vi "Execute.vi"(8 "error in":errorcluster, 11 "O3 Valve Step in":refnum<class "O3 Valve Step.lvclass">) -> (0 "error out":errorcluster, 1 "Next Step?":bool, 2 "MSG":string, 3 "O3 Valve Step out":refnum<class "O3 Valve Step.lvclass">)   [LabVIEW 2016, in "Controller.lvlib" / "O3 Valve Step.lvclass"]
uses:
  O3 Valve Step.lvclass
  C:/Program Files (x86)/National Instruments/LabVIEW 2016/vi.lib/MSR Consulting, LLC/General Reuse/Sequence/STEPS/LEAVES/Switch/Switch Step.lvclass
  Messages/Update O3 Valve State MSG/Update O3 Valve State MSG.lvclass
  G:/sw_repo/For Builds/Nicholas/Controller/Messages/Generic Boolean MSG/Generic Boolean Message.lvclass
  C:/Program Files (x86)/National Instruments/LabVIEW 2016/vi.lib/ActorFramework/Message/Message.lvclass
  Messages/Generic Boolean MSG/Generic Boolean Message.lvclass/Generic Boolean Message.ctl
  <vilib>/ActorFramework/Message Enqueuer/Message Enqueuer.lvclass/Message Enqueuer.ctl
  Messages/Generic Boolean MSG/Write Bool.vi
  <vilib>/ActorFramework/Message Priority Queue/Priority Enqueue.vi
  gController.lvclass
  <vilib>/ActorFramework/Message Enqueuer/Message Enqueuer.lvclass
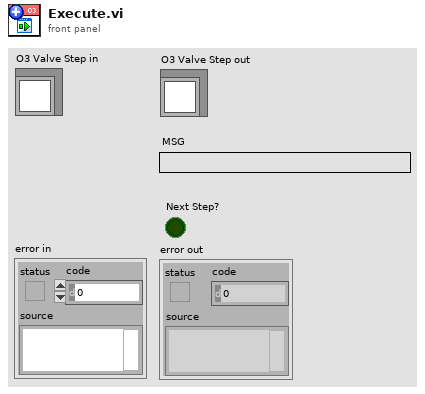
[diagram p1: front panel]
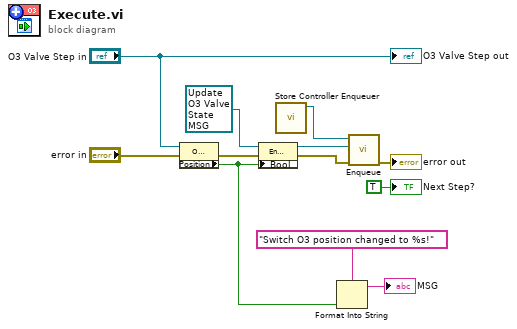
[diagram p0: block diagram]
diagram:
  n1 = property class="O3 Valve Step.lvclass"(reference="O3 Valve Step in", error in="error in") -> (error out=w7:errorcluster, "Position"=w2:bool)  [unwired: 1 out]
  n2 = property class="Enable Compressor MSG"(reference=refnum<class "Update O3 Valve State MSG.lvclass"> refnum ("Controller.lvlib:Enable Compressor MSG"), error in=w7, "Bool"=w2) -> (reference out=w10:refnum<class "Update O3 Valve State MSG.lvclass">, error out=w6:errorcluster)
  n3 = call "Store Controller Enqueuer.vi"() -> ("Controller Enqueuer Out"=w11:refnum<class "Message Enqueuer.lvclass">)  [unwired: 11 in]
  n4 = Format Into String(format string="Switch O3 position changed to %s!" ("MSG 2"), w2) -> (resulting string=→"MSG":string)  [unwired: 2 in, 1 out]
  n5 = call <vilib>:"Enqueue.vi"("error in (no error)"=w6, "Message"=w10, "Message Enqueuer in"=w11) -> ("error out"=→"error out":errorcluster)  [unwired: 7 in, 1 out]
  "O3 Valve Step out" <- "O3 Valve Step in"
  "Next Step?" <- TRUE ("Next Step?")
